vi "MCSMain.vi"(0 "MCSSelectTrigger":T1, 2 "delay(ticks)":u32, 5 "nOfBins":u32) -> ()   [LabVIEW 2014]
uses:
  Controls/MCSselectTrigger.ctl
  <vilib>/Platform/TimedLoop/XDataNode/timing_clust.ctl
  <vilib>/Platform/TimedLoop/XDataNode/nitl_modes.ctl
  <vilib>/Platform/TimedLoop/XDataNode/wakeup.ctl
  <vilib>/rvi/Emulation/niFpgaSctlEmulationGetInTimedLoop.vi
  <vilib>/rvi/Emulation/niFpgaEmulationReportErrorSimple.vi
  <vilib>/rvi/Emulation/niFpgaGetClockAttributes.vi
  <vilib>/rvi/Emulation/niFpgaCriticalErrorInLSC.vi
  Sequencer/sequencerGlobVars.vi
  <vilib>/rvi/eio/common/nirviEmuTemplateMethod_errors.vi
  <vilib>/rvi/Emulation/niFpgaProcessEmulError.vi
  <vilib>/rvi/interface/RandomDataEmulation/niFpgaRandomDataHandleErrors.vi
  <vilib>/Platform/TimedLoop/XDataNode/XDataNode.xnode
  <vilib>/eio/EIONode/EIONode.xnode
  <vilib>/rvi/DataTransferAndStorage/Container/XNode/niFpgaContainer.xnode
  <vilib>/rvi/interface/RandomDataEmulation/nirviRandomDataFpgaReadWriteTemplate.vi
  <vilib>/Platform/TimedLoop/XDataNode/XDNodeRunTimeDep.lvlib
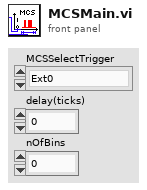
[diagram p1: front panel]
types:
  T1 = typedef "MCSselectTrigger.ctl" = enum8{"Ext0", "Ext1", "Ext2", "Ext3", "Ext4", "Ext5", "Ext6", "Ext7", "Int0", "Int1", "Int2", "Int3", "Int4", "Int5", "Int6", "Int7"}
  T2 = typedef "XDNodeRunTimeDep.lvlib/timing_clust.ctl" = cluster{"Expected End [f-1]":u64, "Actual End [f-1]":u64, "Finished Late? [f-1]":bool, "Expected End [i-1]":u64, "Actual End [i-1]":u64, "Finished Late? [i-1]":bool, "Expected Start [i]":u64, "Actual Start [i]":u64, "Expected Start [f]":u64, "Actual Start [f]":u64, "Source Name":string, "Structure Name":string, "Period":i64, "Deadline":i64, "Offset":i64, "Start":i64, "Priority":i32, "Timeout":i32, "Mode":T3, "Wakeup Reason":T4, "Error":errorcluster, "Source Type":string, "Secondary Source Type":string, "Global End Time":u64, "Global Start Time":u64, "Frame Duration":u64, "Iteration Duration":u64, "Assigned CPU":i32, "I/O Scan Engine Mode":u32}
  T3 = typedef "XDNodeRunTimeDep.lvlib/nitl_modes.ctl" = enum32{"No Change", "Process missed periods, maintain original phase", "Discard missed periods, maintain original phase", "Process missed periods, ignore original phase", "Discard missed periods, ignore original phase"}
  T4 = typedef "XDNodeRunTimeDep.lvlib/wakeup.ctl" = enum32{"Normal", "Aborted", "Asynchronous wakeup", "Timing source error", "Timed loop error", "Timeout"}
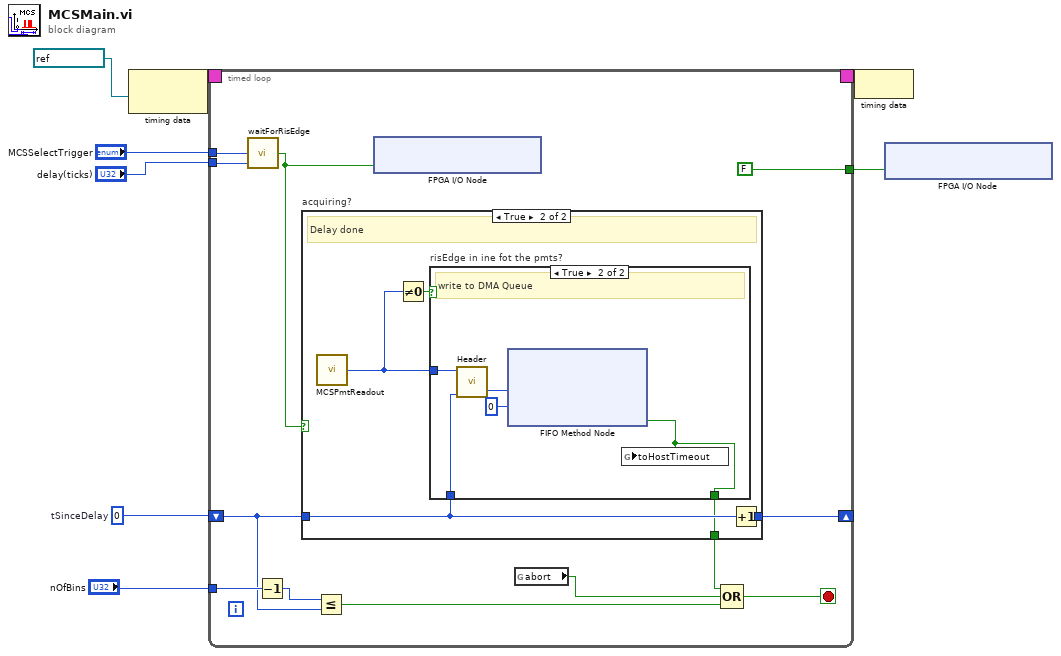
[diagram p0: block diagram]
diagram:
  w4 = u32 0  # tSinceDelay
  n1 = node-c288(refnum<k21> "100MHz" ("Source Name")) -> (w8:T2)
  n2 = timed-loop {
    timing: w8 -> [_]
    timing-out: [_] -> w7
    tunnel: "MCSSelectTrigger" -> [w19]
    shift-right: [w20] -> _
    shift-left: w4 -> [w15]
    tunnel: "delay(ticks)" -> [w18]
    tunnel: "nOfBins" -> [w17]
    tunnel: [FALSE ("result")] -> w1
    stop <- w11 stop-if-true
    n3 = call "waitForRisEdge.vi"("delay(ticks)"=w18, "MCSSelectTrigger"=w19) -> ("out"=w10:bool)  [unwired: 3 in]
    n4 = Decrement(x=w17) -> (x-1=w16:u32)
    n5 = case "acquiring?" shown="True" w10 {
      tunnel: w15 -> [w21 w23]
      tunnel: [w21 w26] -> w20
      tunnel: [_ w22] -> w12
      frame False {
      }
      frame True {
        # "Delay done"
        n6 = call "MCSPmtReadout.vi"() -> ("pmtOut"=w24:u8)  [unwired: 5 in]
        n7 = Not Equal To 0?(x=w24) -> (x != 0?=w25:bool)
        n8 = case "risEdge in ine fot the pmts?" shown="True" w25 {
          tunnel: w24 -> [_ w31]
          tunnel: w23 -> [_ w29]
          tunnel: [_ w27] -> w22
          frame False {
          }
          frame True {
            # "write to DMA Queue"
            n9 = call "Header.vi"("23BitData"=w29, "8BitHead"=w31) -> ("32BitOutput"=w30:u32)  [unwired: 3 in]
            n10 = xnode ("FIFO Method Node")("Element"=w30, "Timeout"=0) -> ("Timed Out?"=w27:bool)  [unwired: 1 in, 1 out]
            n11 = global write "sequencerGlobVars.vi" "toHostTimeout"(w27) -> ()
          }
        }
        n12 = Increment(x=w23) -> (x+1=w26:u32)
      }
    }
    n13 = Less Or Equal?(x=w16, y=w15) -> (x <= y?=w14:bool)
    n14 = xnode "FPGA I/O Node"("MCSScanFlagDio9Con1"=w10) -> ()  [unwired: 1 in, 1 out]
    n15 = global read "sequencerGlobVars.vi" "abort"() -> (w13:bool)
    n16 = Compound Arithmetic op=OR(w12, w13, w14) -> (w11:bool)
  }
  n17 = node-c288(w7) -> ()
  n18 = xnode "FPGA I/O Node"("MCSScanFlagDio9Con1"=w1) -> ()  [unwired: 1 in, 1 out]
